vi "Handle Error.vi"(8 "error in (no error)":errorcluster caption="错误输入（无错误）", 11 "Input Operator in":refnum<class "ControlPanel.lvclass"> caption="操作者输入") -> (0 "error out":errorcluster caption="错误输出", 2 "stop actor?":bool=TRUE caption="停止操作者？", 3 "Input Operator out":refnum<class "ControlPanel.lvclass"> caption="操作者输出")   [LabVIEW 2014, in "ControlPanel.lvlib" / "ControlPanel.lvclass"]
doc: "(<B>Filename</B>: Actor Framework.lvlib:Actor.lvclass:Handle Error.vi)\n\nDefines how the actor handles an error that occurred while processing a message. By default, this method does nothing except stop the actor."
uses:
  ControlPanel.lvclass
  <vilib>/ActorFramework/Actor/Actor.lvclass
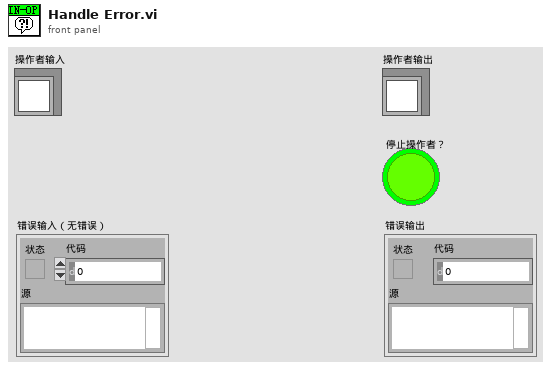
[diagram p1: front panel]
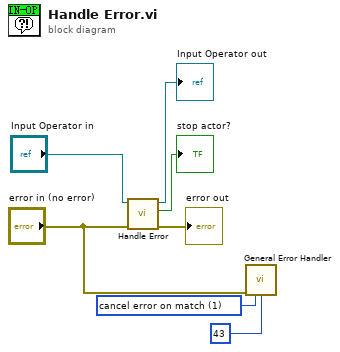
[diagram p0: block diagram]
diagram:
  w2 = 1 items=["no exception", "cancel error on match", "set error on match"] ("[exception action] (none:0)")
  n1 = call-parent "Handle Error.vi"("error in (no error)"="error in (no error)", "Actor in"="Input Operator in") -> ("error out"=→"error out":errorcluster, "stop actor?"=→"stop actor?":bool, "Actor out"=→"Input Operator out":refnum<class "ControlPanel.lvclass">)  [unwired: 7 in]
  n2 = call <vilib>:"General Error Handler.vi"("error in (no error)"="error in (no error)", "[exception action] (none:0)"=w2, "[exception code]"=43) -> ()  [unwired: 8 in, 5 out]
